vi "ViewLayer.vi"(7 "Add to Undo?":bool, 8 "error in (no error)":errorcluster, 11 "Data in":T1={"Class"={"Ants"=refnum, "Layer"=refnum, "Templates"=refnum, "Icon"=refnum, "Glyph"=refnum, "Settings"=refnum, "Tools"=refnum, "History"=refnum}, "Ref"={"Add Layer"=refnum, "Remove Layer"=refnum, "Line Text"=[], "Body Text Spec"=refnum, "DNL_Font"=refnum, "glyph path str"=refnum, "templates path str"=refnum, "Arrow Up"=refnum, "Arrow Down"=refnum, "IE VI Ref"=refnum, "Glyphs tree"=refnum, "Templates tree"=refnum, "Layer Icon Text"=refnum, "Layer Template"=refnum, "Body Text"=refnum, "Search Templates"=refnum, "TextMarker"=refnum, "Tab Control"=refnum, "Search Glyphs"=refnum, "Line Color"=refnum, "DNL_Glyphs []"=refnum, "Fill Color"=refnum, "Tools"=refnum, "Icon"=refnum, "Preview"=refnum, "Ants"=refnum, "Terminals"=refnum, "menu reference"=refnum, "LayerNames"=[], "GlyphLoadAnimation"=refnum, "TemplateLoadAnimation"=refnum, "refreshGlyphs"=refnum, "refreshTemplates"=refnum}, "Support"={"AntsRect"={"left"=0, "top"=0, "right"=0, "bottom"=0}, "Mouse Move Coords"={"Horizontal"=0, "Vertical"=0}, "Mouse Down Coords"={"Horizontal"=0, "Vertical"=0}, "Temp Coord"={"Horizontal"=0, "Vertical"=0}, "Action"=enum."Default", "Edge Color"=4914962, "Fill Color"=16860, "Mouse Down?"=FALSE, "Draft Mode?"=FALSE, "Temp Icon"=bytes[3102], "CTRL Pressed"=FALSE, "Move Selection?"=FALSE, "AntsRect Orig"={"left"=0, "top"=0, "right"=0, "bottom"=0}, "Text"="", "TM Set?"=FALSE, "Mouse inside icon?"=FALSE, "Tool (old value)"=0, "Pencil Move Color"=0, "Swap Colors?"=FALSE, "Shift pressed?"=FALSE}}) -> (0 "error out":errorcluster, 3 "Data out":T1={"Class"={"Ants"=refnum, "Layer"=refnum, "Templates"=refnum, "Icon"=refnum, "Glyph"=refnum, "Settings"=refnum, "Tools"=refnum, "History"=refnum}, "Ref"={"Add Layer"=refnum, "Remove Layer"=refnum, "Line Text"=[], "Body Text Spec"=refnum, "DNL_Font"=refnum, "glyph path str"=refnum, "templates path str"=refnum, "Arrow Up"=refnum, "Arrow Down"=refnum, "IE VI Ref"=refnum, "Glyphs tree"=refnum, "Templates tree"=refnum, "Layer Icon Text"=refnum, "Layer Template"=refnum, "Body Text"=refnum, "Search Templates"=refnum, "TextMarker"=refnum, "Tab Control"=refnum, "Search Glyphs"=refnum, "Line Color"=refnum, "DNL_Glyphs []"=refnum, "Fill Color"=refnum, "Tools"=refnum, "Icon"=refnum, "Preview"=refnum, "Ants"=refnum, "Terminals"=refnum, "menu reference"=refnum, "LayerNames"=[], "GlyphLoadAnimation"=refnum, "TemplateLoadAnimation"=refnum, "refreshGlyphs"=refnum, "refreshTemplates"=refnum}, "Support"={"AntsRect"={"left"=0, "top"=0, "right"=0, "bottom"=0}, "Mouse Move Coords"={"Horizontal"=0, "Vertical"=0}, "Mouse Down Coords"={"Horizontal"=0, "Vertical"=0}, "Temp Coord"={"Horizontal"=0, "Vertical"=0}, "Action"=enum."Default", "Edge Color"=4914962, "Fill Color"=16860, "Mouse Down?"=FALSE, "Draft Mode?"=FALSE, "Temp Icon"=bytes[3102], "CTRL Pressed"=FALSE, "Move Selection?"=FALSE, "AntsRect Orig"={"left"=0, "top"=0, "right"=0, "bottom"=0}, "Text"="", "TM Set?"=FALSE, "Mouse inside icon?"=FALSE, "Tool (old value)"=0, "Pencil Move Color"=0, "Swap Colors?"=FALSE, "Shift pressed?"=FALSE}})   [LabVIEW 2020]
uses:
  Class/Ants/Ants.lvclass
  Class/FakedArray/FakedArray.lvclass
  vi.lib/LabVIEW Icon API/lv_icon/Classes/Icon/Icon.lvclass
  Class/Icon Library/Glyph.lvclass
  Class/Settings/Settings.lvclass
  Class/Tools/Tools Paint.lvclass
  vi.lib/LabVIEW Icon API/lv_icon/Classes/Layer/Layer.lvclass
  History/History.lvlib
  <vilib>/Utility/miscctls.llb/LVPoint32TypeDef.ctl
  Controls/SupportClass_Action.ctl
  vi.lib/LabVIEW Icon API/lv_icon/Controls/IEColor.ctl
  Controls/Support Cluster.ctl
  lv_icon.lvlib
  Controls/References Cluster.ctl
  Controls/IE Classes.ctl
  Controls/Global Data.ctl
  History/History/History.lvclass
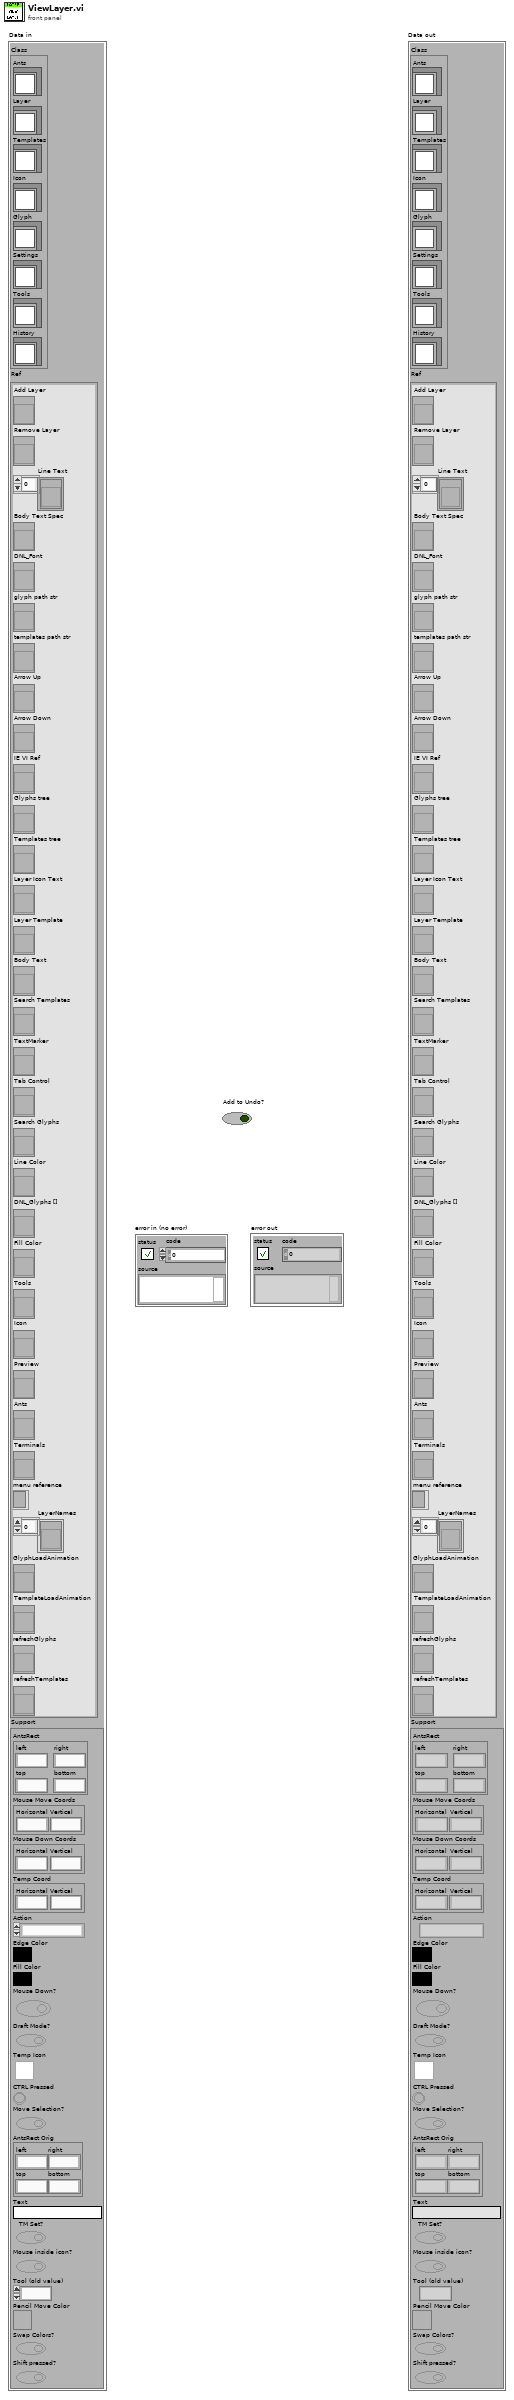
[diagram p1: front panel]
types:
  T1 = typedef "lv_icon.lvlib/Global Data.ctl" = cluster{"Class":T2, "Ref":T3, "Support":T4}
  T2 = typedef "lv_icon.lvlib/IE Classes.ctl" = cluster{"Ants":refnum<class "Ants.lvclass">, "Layer":refnum<class "FakedArray.lvclass">, "Templates":refnum<class "FakedArray.lvclass">, "Icon":refnum<class "Icon.lvclass">, "Glyph":refnum<class "Glyph.lvclass">, "Settings":refnum<class "Settings.lvclass">, "Tools":refnum<class "Tools Paint.lvclass">, "History":refnum<class "History.lvclass">}
  T3 = typedef "lv_icon.lvlib/References Cluster.ctl" = cluster{"Add Layer":refnum<vi>, "Remove Layer":refnum<vi>, "Line Text":refnum<vi>[], "Body Text Spec":refnum<vi>, "DNL_Font":refnum<vi>, "glyph path str":refnum<vi>, "templates path str":refnum<vi>, "Arrow Up":refnum<vi>, "Arrow Down":refnum<vi>, "IE VI Ref":refnum<vi>, "Glyphs tree":refnum<vi>, "Templates tree":refnum<vi>, "Layer Icon Text":refnum<vi>, "Layer Template":refnum<vi>, "Body Text":refnum<vi>, "Search Templates":refnum<vi>, "TextMarker":refnum<vi>, "Tab Control":refnum<vi>, "Search Glyphs":refnum<vi>, "Line Color":refnum<vi>, "DNL_Glyphs []":refnum<vi>, "Fill Color":refnum<vi>, "Tools":refnum<vi>, "Icon":refnum<vi>, "Preview":refnum<vi>, "Ants":refnum<vi>, "Terminals":refnum<vi>, "menu reference":refnum<k9>, "LayerNames":refnum<vi>[], "GlyphLoadAnimation":refnum<vi>, "TemplateLoadAnimation":refnum<vi>, "refreshGlyphs":refnum<vi>, "refreshTemplates":refnum<vi>}
  T4 = typedef "lv_icon.lvlib/Support Cluster.ctl" = cluster{"AntsRect":cluster{"left":i16, "top":i16, "right":i16, "bottom":i16}, "Mouse Move Coords":T5, "Mouse Down Coords":T5, "Temp Coord":T5, "Action":T6, "Edge Color":T7, "Fill Color":T7, "Mouse Down?":bool, "Draft Mode?":bool, "Temp Icon":picture, "CTRL Pressed":bool, "Move Selection?":bool, "AntsRect Orig":cluster{"left":i16, "top":i16, "right":i16, "bottom":i16}, "Text":string, "TM Set?":bool, "Mouse inside icon?":bool, "Tool (old value)":u32, "Pencil Move Color":u32, "Swap Colors?":bool, "Shift pressed?":bool}
  T5 = typedef "LVPoint32TypeDef.ctl" = cluster{"Horizontal":i32, "Vertical":i32}
  T6 = typedef "SupportClass_Action.ctl" = enum16{"Default", "Move Selection", "Glyph Library", "Tool"}
  T7 = typedef "IEColor.ctl" = u32
  T8 = cluster{"Pointer Absolute":i32, "Cluster Refnum":refnum<vi>, "# Rows":i32, "# Cols":i32, "Scrollbar Position":i32, "Pointer Absolute Row":i32, "Pointer Absolute Col":i32}
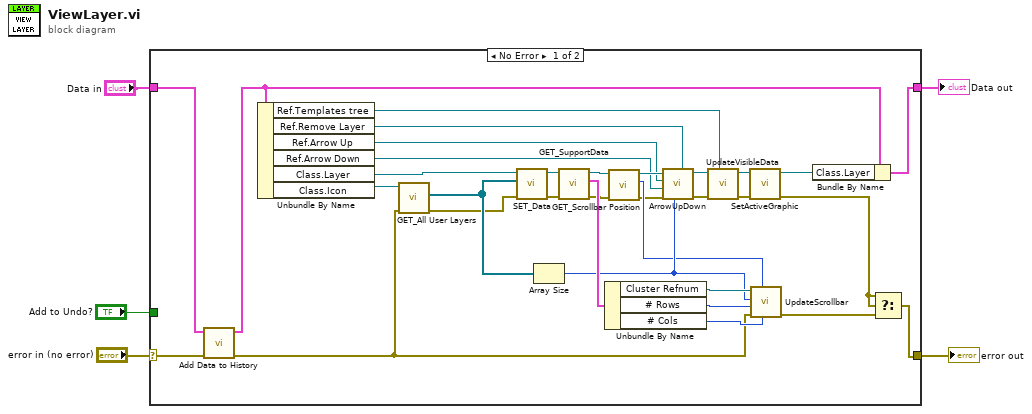
[diagram p0: block diagram]
diagram:
  n1 = case shown="No Error" "error in (no error)" {
    selector: "error in (no error)" -> [w38 w40]
    tunnel: [w20 w40] -> w4
    tunnel: "Add to Undo?" -> [_ _]
    tunnel: "Data in" -> [w16 w39]
    tunnel: [w17 w39] -> w1
    frame No Error {
      n2 = call "Add Data to History.vi"("error in"=w38, "Data in"=w16) -> ("error out"=w12:errorcluster, "Data out"=w15:T1)  [unwired: 1 in, 7 out]
      n3 = Unbundle By Name(w15) -> ("Ref.Templates tree"=w7:refnum<vi>, "Ref.Remove Layer"=w6:refnum<vi>, "Ref.Arrow Up"=w8:refnum<vi>, "Ref.Arrow Down"=w9:refnum<vi>, "Class.Layer"=w19:refnum<class "FakedArray.lvclass">, "Class.Icon"=w14:refnum<class "Icon.lvclass">)
      n4 = call-dynamic "GET_All User Layers.vi"("error in (no error)"=w12, "Icon.lvclass in"=w14) -> ("error out"=w11:errorcluster, "User Layer"=w13:refnum<class "Layer.lvclass">[])  [unwired: 8 out]
      n5 = call-dynamic "SET_Data.vi"("error in (no error)"=w11, "Data"=w13, "FakedArray in"=w19) -> ("error out"=w30:errorcluster, "FakedArray out"=w29:refnum<class "FakedArray.lvclass">)  [unwired: 7 out]
      n6 = Array Size(array=w13) -> (size(s)=w28:i32)
      n7 = call-dynamic "GET_SupportData.vi"("error in (no error)"=w30, "FakedArray in"=w29) -> ("error out"=w27:errorcluster, "Cluster"=w31:T8, "FakedArray out"=w26:refnum<class "FakedArray.lvclass">)  [unwired: 7 out]
      n8 = Unbundle By Name(w31) -> ("Cluster Refnum"=w32:refnum<vi>, "# Rows"=w33:i32, "# Cols"=w24:i32)
      n9 = call-dynamic "GET_Scrollbar Position.vi"("error in (no error)"=w27, "FakedArray.lvclass in"=w26) -> ("error out"=w23:errorcluster, "Scrollbar Position"=w25:i32, "FakedArray.lvclass out"=w22:refnum<class "FakedArray.lvclass">)  [unwired: 7 out]
      n10 = call "ArrowUpDown.vi"("Remove Layer"=w6, "# Layers"=w28, "error in (no error)"=w23, "Arrow Down"=w9, "Arrow Up"=w8, "FakedArray in"=w22) -> ("error out"=w35:errorcluster, "FakedArray out"=w34:refnum<class "FakedArray.lvclass">)  [unwired: 4 out]
      n11 = call-dynamic "UpdateVisibleData.vi"("Templates tree"=w7, "error in (no error)"=w35, "FakedArray in"=w34) -> ("error out"=w36:errorcluster, "FakedArray out"=w37:refnum<class "FakedArray.lvclass">)  [unwired: 2 in, 5 out]
      n12 = call-dynamic "SetActiveGraphic.vi"("error in (no error)"=w36, "FakedArray in"=w37) -> ("error out"=w10:errorcluster, "FakedArray out"=w18:refnum<class "FakedArray.lvclass">)  [unwired: 4 in, 4 out]
      n13 = call "UpdateScrollbar.vi"("# Cols"=w24, "Value Scrollbar"=w25, "error in"=w12, "#Rows"=w33, "# Elements"=w28, "Cluster Refnum"=w32) -> ("error out"=w21:errorcluster)  [unwired: 5 out]
      n14 = Bundle By Name(cluster=w15, "Class.Layer"=w18) -> (w17:T1)
      n15 = Select(t=w10, s=w10, f=w21) -> (s? t:f=w20:errorcluster)
    }
    frame Error {
    }
  }
  "error out" <- w4
  "Data out" <- w1
